vi "semantic_camera.vi"(0 "Camera configuration":string=" {\n     \"type\": \"SemanticCamera\",\n     \"listen_port\": 8013,\n     \"location\": {\n       \"x\": 0.0,\n       \"y\": 0.0,\n       \"z\": 250.0\n     },\n     \"rotation\": {\n       \"pitch\": 0.0,\n       \"yaw\": 0.0,\n       \"roll\": 0.0\n     },\n     \"stream_dimensions\": {\n       \"x\": 512.0,\n       \"y\": 512.0\n     },\n   \"dynamic_range\": 1.0,\n  \t\"fov\": 60.0,\n   \"camera_matrix\": [\n        [433.0, 0.0,   256.0],\n        [0.0,   433.0, 256.0],\n        [0.0,   0.0,   1.0]\n    ],\t\n \t\"min_shutter\": 0.0005,\n  \t\"max_shutter\": 0.0014,\n   \"motion_blur_bias\": 0.1,\n   \"white_balance\": 0.0,\n   \"white_balance_temp_offset\": 0,\n   \"exposure_compensation\": -1.0,\n   \"image_noise_bias\": 0.05,\n   \"channels\" : \"gray\",\n   \"ray_tracing\":{\n        \"enable_ray_tracing\": false\n     },\n   \"annotation\": {\n      \"include_annotation\": false,\n      \"desired_tags\": [\n        \"traffic_sign\", \"vehicle\"\n      ],\n      \"include_lanes\": true,\n\t\t    \"lane_sampling_distance\": 15000.0,\n     \t\"lane_sampling_frequency\": 100.0,\n\t\t    \"lane_subsampling\": 10.0,\n      \"far_plane\": 10000.0,\n      \"include_tags\": true,\n      \"include_obb\": false,\n      \"cull_partial_frame\":false,\n      \"debug_draw\":false\n    },\n    \"max_distance\":50000.0,\n    \"channel_depth\": 1\n }\n", 3 "Error In":errorcluster) -> (4 "Camera configuration":string, 6 "Image":picture, 7 "Raw data":u8[](array[numeric]), 8 "Annotation data":string, 9 "Error Out":errorcluster)   [LabVIEW 2019, in "Lib_Simx.lvlib"]
doc: "Configures and reads the data stream for a Semantic Camera sensor and outputs a picture of the specified size on the Camera configuration."
uses:
  Lib_Simx.lvlib
  tools/simx_common.vi
  controls/Header.ctl
panel:
  out "Header":T1 {"game_time" format="%_10g"}
  in  "Show Annotation":bool
  # "Note: set annotation settings in camera configuration json"
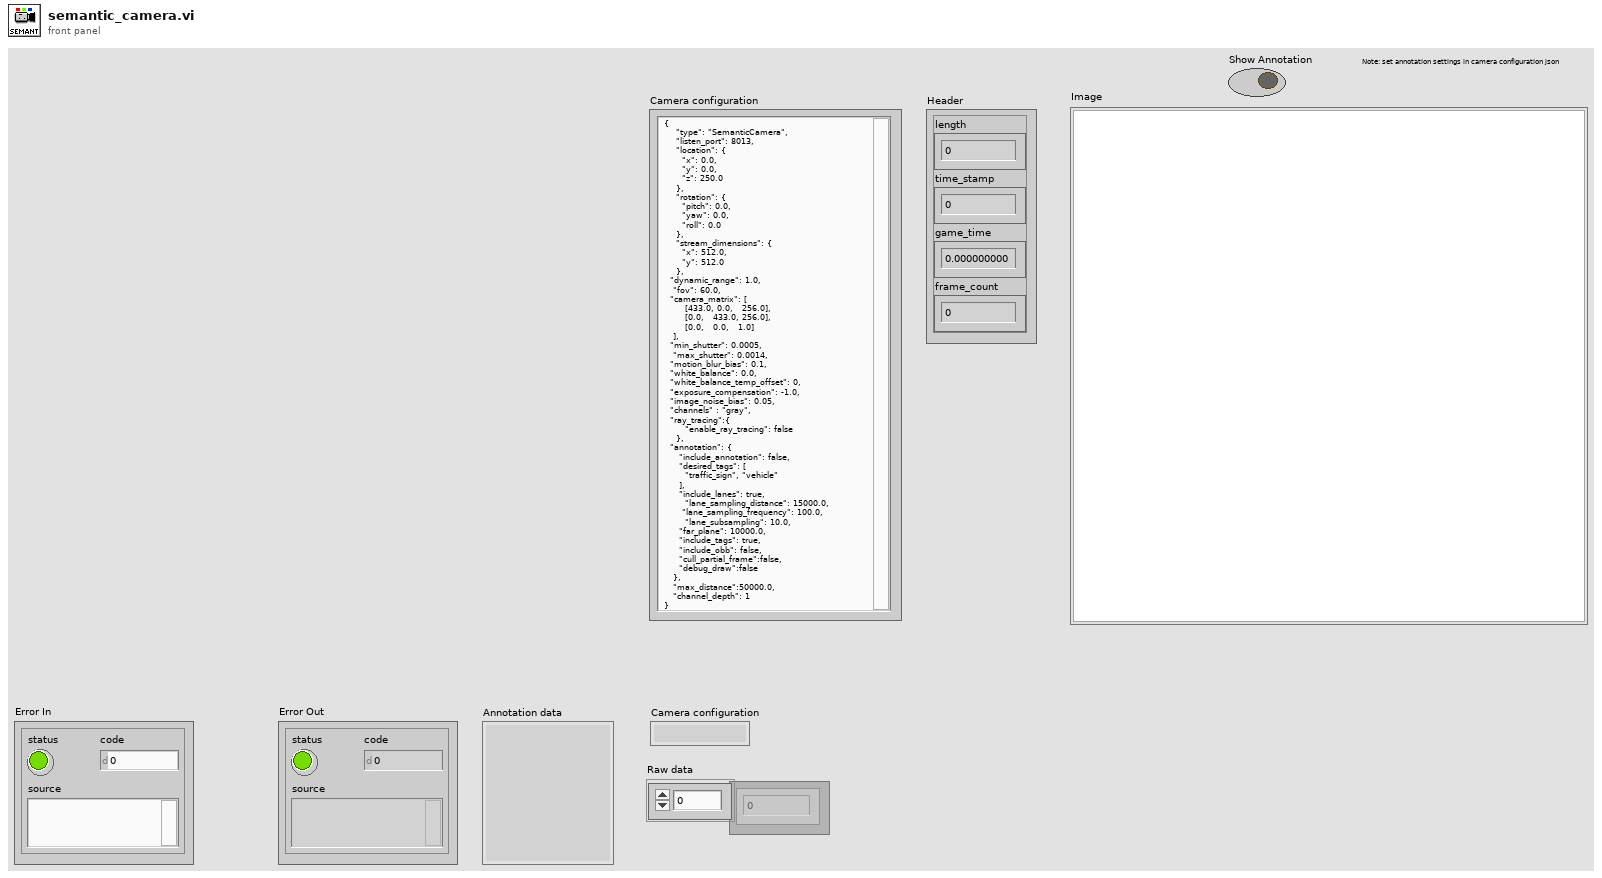
[diagram p1: front panel]
types:
  T1 = typedef "Lib_Simx.lvlib/Header.ctl" = cluster{"length":u32, "time_stamp":u32, "game_time":sgl, "frame_count":u32}
  T2 = typedef "Lib_Simx.lvlib/simx_connection.ctl" = cluster{"Config":T3, "Connections":T6, "Map":cluster{"lanes":cluster{"x":dbl[], "y":dbl[], "z":dbl[]}, "StartPosition":cluster{"start_points":T7, "StartRotation":dbl[], "StartLocation":dbl[]}, "Draw Map Size":T8, "DrawArea":cluster{"min_Y":dbl, "min_X":dbl, "Scale X":dbl, "Scale Y":dbl}, "Map":picture, "Map Geojson":string}}
  T3 = typedef "Lib_Simx.lvlib/config.ctl" = cluster{"Trajectory":T4, "Weather":T5}
  T4 = typedef "Lib_Simx.lvlib/trajectory.ctl" = cluster{"Number of frames":i32, "Frame number":i32, "Trajectory":string}
  T5 = typedef "Lib_Simx.lvlib/weather.ctl" = cluster{"id":string}
  T6 = typedef "Lib_Simx.lvlib/connections.ctl" = cluster{"Simulator Connection":refnum<k5>, "server_ip":string, "Port":i32, "Sensor connections":refnum<k5>[]}
  T7 = typedef "Lib_Simx.lvlib/start_points.ctl" = cluster{"locations":dbl[][], "rotations":dbl[][], "type":string[]}
  T8 = typedef "LVBoundsTypeDef.ctl" = cluster{"Width":u32, "Height":u32}
  T9 = typedef "Lib_Simx.lvlib/sensor_sample.ctl" = cluster{"Header":T1, "data out":string}
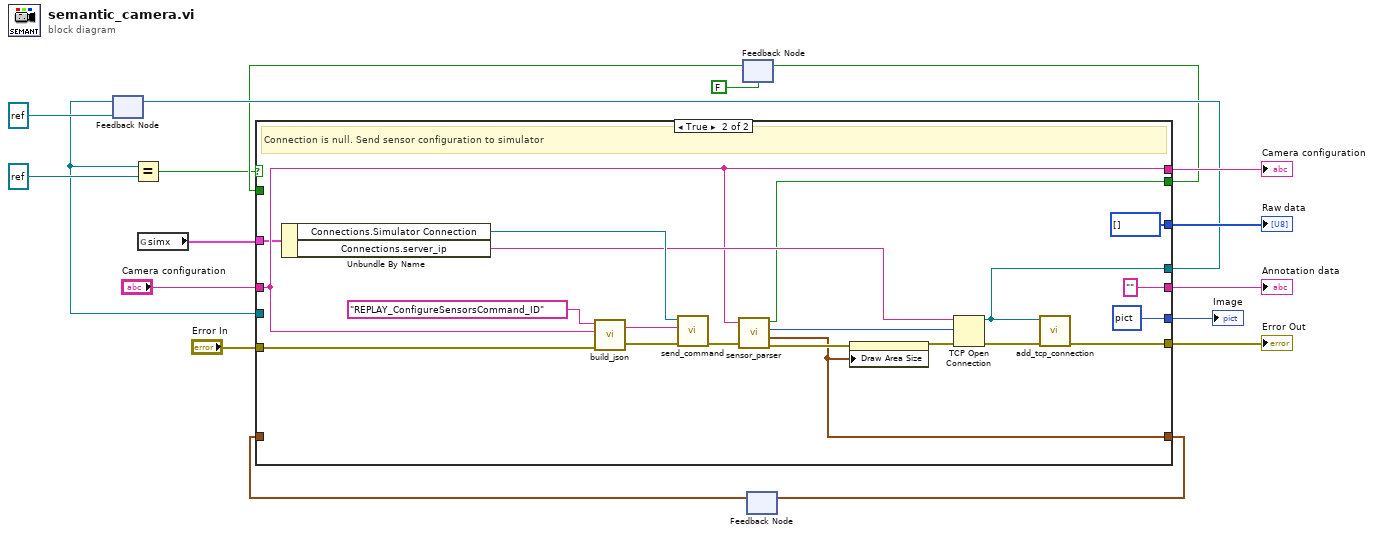
[diagram p0: block diagram]
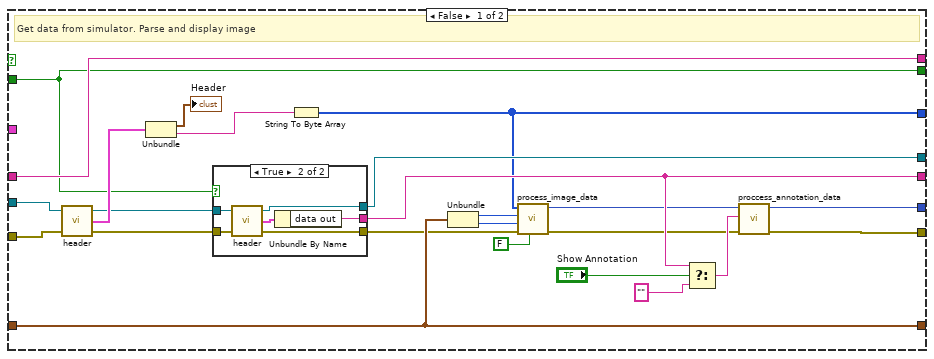
[diagram p2: hidden frame]
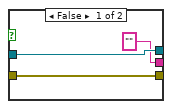
[diagram p3: hidden frame]
diagram:
  n1 = feedback #1(refnum<k5> refnum ("camera_connection")) -> (w11:refnum<k5>)
  n2 = Equal?(x=w11, y=refnum<k5> refnum ("null connection")) -> (x = y?=w1:bool)
  n3 = global read "simx_common.vi" "simx"() -> (w15:T2)
  n4 = feedback #2(FALSE) -> (w2:bool)
  n5 = feedback #3() -> (w9:cluster{"x dimension":i32, "y dimension":i32})  [unwired: 1 in]
  n6 = case shown="True" w1 {
    tunnel: [w35 w52] -> w12
    tunnel: "Camera configuration" -> [w37 w56]
    tunnel: [w27 w54] -> w4
    tunnel: w11 -> [w40 _]
    tunnel: "Error In" -> [w39 w62]
    tunnel: w9 -> [w38 _]
    tunnel: [w34 picture data[5B] ("new picture")] -> w6
    tunnel: [w38 w59] -> w10
    tunnel: [w23 u8[] [] ("unsigned byte array")] -> w5
    tunnel: [w37 w56] -> w8
    tunnel: [w36 w58] -> w3
    tunnel: w2 -> [w36 _]
    tunnel: [w33 "" ("data out")] -> w7
    tunnel: w15 -> [_ w55]
    frame False {
      # "Get data from simulator. Parse and display image"
      n7 = call "header.vi"("error in"=w39, "TCP Network Connection in"=w40) -> ("error out"=w24:errorcluster, "Sensor sample"=w41:T9, "TCP Network Connection out"=w31:refnum<k5>)  [unwired: 1 in]
      n8 = Unbundle(w41) -> ("Header"=→"Header":T1, "data out"=w42:string)
      n9 = case shown="True" w36 {
        tunnel: w31 -> [w45 w51]
        tunnel: [w45 w50] -> w27
        tunnel: w24 -> [w43 w49]
        tunnel: ["" ("data out") w47] -> w33
        tunnel: [w43 w46] -> w26
        frame False {
        }
        frame True {
          n10 = call "header.vi"("error in"=w49, "TCP Network Connection in"=w51) -> ("error out"=w46:errorcluster, "Sensor sample"=w48:T9, "TCP Network Connection out"=w50:refnum<k5>)  [unwired: 1 in]
          n11 = Unbundle By Name(w48) -> ("data out"=w47:string)
        }
      }
      n12 = String To Byte Array(string=w42) -> (unsigned byte array=w23:u8[])
      n13 = Unbundle(w38) -> ("x dimension"=w22:i32, "y dimension"=w21:i32)
      n14 = call "process_image_data.vi"("RGBA"=FALSE, "error in"=w26, "y"=w21, "x"=w22, "Raw data"=w23) -> ("error out"=w25:errorcluster, "Image"=w20:picture)  [unwired: 3 in]
      n15 = Select(t=w33, s="Show Annotation", f="") -> (s? t:f=w28:string)
      n16 = call "proccess_annotation_data.vi"("error in"=w25, "Annotation Data"=w28, "Image in"=w20) -> ("error out"=w35:errorcluster, "Image out"=w34:picture)  [unwired: 2 in, 1 out]
    }
    frame True {
      # "Connection is null. Send sensor configuration to simulator"
      n17 = Unbundle By Name(w55) -> ("Connections.Simulator Connection"=w65:refnum<k5>, "Connections.server_ip"=w63:string)
      n18 = call "build_json.vi"("error in"=w62, "Message"=w56, "Command_ID"="REPLAY_ConfigureSensorsCommand_ID") -> ("error out"=w69:errorcluster, "JSON Out"=w70:string)  [unwired: 1 in]
      n19 = call "send_command.vi"("error in"=w69, "JSON Command"=w70, "TCP Network Connection in"=w65) -> ("error out"=w61:errorcluster)  [unwired: 1 in, 3 out]
      n20 = call "sensor_parser.vi"("Sensor configuration"=w56, "error in"=w61) -> ("include_annotation"=w58:bool, "Port out"=w57:u16, "Stream dimensions"=w59:cluster{"x dimension":i32, "y dimension":i32}, "error out"=w60:errorcluster)  [unwired: 1 in]
      n21 = property on="Image" class="Pict"(error in=w60, "Draw Area Size"=w59) -> (error out=w64:errorcluster)  [unwired: 1 in, 1 out]
      n22 = TCP Open Connection(address=w63, remote port or service name=w57, error in (no error)=w64) -> (connection ID=w54:refnum<k5>, error out=w53:errorcluster)  [unwired: 2 in]
      n23 = call "add_tcp_connection.vi"("error in"=w53, "Sensor connection"=w54) -> ("error out"=w52:errorcluster)  [unwired: 5 in]
    }
  }
  "Error Out" <- w12
  "Image" <- w6
  "Raw data" <- w5
  "Camera configuration" <- w8
  "Annotation data" <- w7
  n24 = feedback-in #1(w4) -> ()
  n25 = feedback-in #2(w3) -> ()
  n26 = feedback-in #3(w10) -> ()
